vi "Meas Dig Frequency-Low Freq 1 Ctr.vi"() -> ()   [LabVIEW 2010]
doc: "I. Description:\nThis example demonstrates how to measure frequency using one counter on a Counter Input Channel. The Edge, Minimum Value and Maximum Value are all configurable. \n\nThis example shows how to measure frequency on the counter's default input terminal (refer to section IV, I/O Connections Overview, below for more information), but could easily be expanded to measure frequency on any PFI, RTSI, or internal signal. Additionally, this example could be extended to measure frequency with two counters for different frequency and quantization error requirements.\n\nII. Instructions for Running:\n1. Select the Physical Channel which corresponds to the counter you want to measure frequency on the DAQ device.\n2. Enter the measurement Edge to specify the edge on which you want the counter to start measuring. Enter the Maximum and Minimum Value to specify the range or your unknown frequency. Additionally, you can change the input terminal where the frequency is measured using the channel property node.\nNote: It is important to set the Maximum and Minimum Values of your unknown frequency as accurately as possible so the best internal timebase can be chosen to minimize measurement error. The default values specify a range that can be measured by the counter using the 20MhzTimebase. Use the Gen Dig Pulse Train-Continuous example to verify that you are measuring correctly on the DAQ device.\n\nIII. Block Diagram Steps:\n1. Create a Counter Input channel to Frequency. The Edge parameter is used to determine if the counter will begin measuring on a rising or falling edge. It is important to set the Maximum and Minimum Values of your unknown signal as accurately as possible so the best internal timebase can be chosen to minimize measurement error. The default values specify a range that can be measured by the counter using the 20MhzTimebase.\n2. Call the Read VI to return the next frequency measurement. Set a timeout so an error is returned if a period is not returned in the specified time limit.\n3. Call the Clear Task VI to clear the Task \n4. Use the popup dialog box to display an error if any.\n\nIV. I/O Connections Overview:\nThe counter will measure frequency on the input terminal of the counter specified in the Physical Channel I/O control. \n\nFor more information on the default counter input and output terminals for your device, open the NI-DAQmx Help, and refer to Counter Signal Connections found under the Device Considerations book in the table of contents."
uses:
  <vilib>/Utility/error.llb/DialogType.ctl
  <vilib>/DAQmx/read.llb/DAQmx Read (Counter DBL 1Chan 1Samp).vi
  <vilib>/DAQmx/create/channels.llb/DAQmx Create Channel (CI-Frequency).vi
  <vilib>/daqmx/miscellaneous.llb/DAQmx Fill In Error Info.vi
panel:
  in  "Minimum Value (Hz)":dbl=1.192093 format="%0.6f"
  in  "Maximum Value (Hz)":dbl=10000000.0 format="%0.6f"
  in  "Edge":i32(ring)=10280 items=["Rising"=10280, "Falling"=10171]
  in  "Counter(s)":tag="Dev1/ctr0" caption="Counter"
  out "Frequency (Hz)":dbl format="%0.9f"
  # "For instructions, select Help>>Show Context Help"
  # "Channel Parameters"
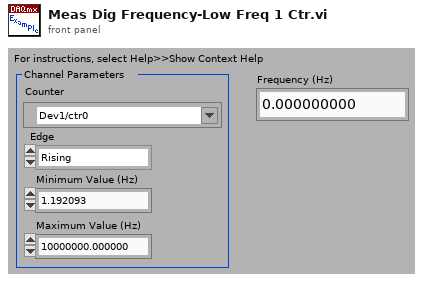
[diagram p1: front panel]
types:
  T1 = typedef "DialogType.ctl" = u16
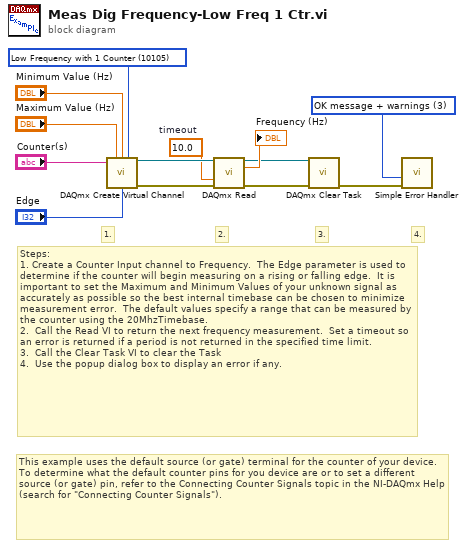
[diagram p0: block diagram]
diagram:
  w4 = T1 3 items=["no dialog", "OK message", "continue or stop message", "OK message + warnings", "continue/stop + warnings"] ("type of dialog (OK msg:1)")
  w5 = 10.0  # timeout
  w11 = 10105 items=["Low Frequency with 1 Counter"=10105, "High Frequency with 2 Counters"=10157, "Large Range with 2 Counters"=10205] ("measurement method")
  # "This example uses the default source (or gate) terminal for the counter of your device.  To determine what the default counter pins for you device are or to set a different source (or gate) pin, refer to the Connecting Counter Signals topic in the NI-DAQmx Help (search for \"Connecting Counter Signals\")."
  # "3."
  # "2."
  # "Steps: \n1. Create a Counter Input channel to Frequency.  The Edge parameter is used to determine if the counter will begin measuring on a rising or falling edge.  It is important to set the Maximum and Minimum Values of your unknown signal as accurately as possible so the best internal timebase can be chosen to minimize measurement error.  The default values specify a range that can be measured by the counter using the 20MhzTimebase.\n2.  Call the Read VI to return the next frequency measurement.  Set a timeout so an error is returned if a period is not returned in the specified time limit.\n3.  Call the Clear Task VI to clear the Task \n4.  Use the popup dialog box to display an error if any."
  # "4."
  # "1."
  n1 = call-poly <vilib>:"DAQmx Create Virtual Channel.vi"("maximum value"="Maximum Value (Hz)", "minimum value"="Minimum Value (Hz)", "measurement method"=w11, "counter"="Counter(s)", "starting edge"="Edge") -> ("task out"=w13:refnum<k21>, "error out"=w12:errorcluster)  [unwired: 9 in]
  n2 = call-poly <vilib>:"DAQmx Read.vi"("task/channels in"=w13, "timeout"=w5, "error in"=w12) -> ("task out"=w3:refnum<k21>, "data"=→"Frequency (Hz)":dbl, "error out"=w2:errorcluster)  [unwired: 10 in]
  n3 = call <vilib>:"DAQmx Clear Task.vi"("task in"=w3, "error in"=w2) -> ("error out"=w1:errorcluster)  [unwired: 13 in]
  n4 = call <vilib>:"Simple Error Handler.vi"("type of dialog (OK msg:1)"=w4, "error in (no error)"=w1) -> ()  [unwired: 3 in, 5 out]
